vi "Add Annotation (by index).vi"(0 "FSM in":refnum<class "FSM.Graph.lvclass">, 5 "selectedEdge":i32, 7 "Name":string, 9 "Style":T1, 11 "error in (no error)":errorcluster) -> (4 "FSM out":refnum<class "FSM.Graph.lvclass">, 6 "Changed?":bool, 15 "error out":errorcluster)   [LabVIEW 2015, in "FSM.Graph.lvclass"]
uses:
  FSM.Graph.lvclass
  FSM.Annotation/Annotation Style.ctl
  FSM.Graph.lvclass/FSM.Graph.ctl
  FSM.Edge/FSM.Edge.lvclass
  FSM.Annotation/FSM.Annotation.lvclass
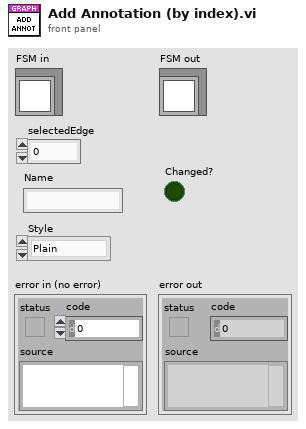
[diagram p1: front panel]
types:
  T1 = typedef "FSM.Annotation.lvclass/Annotation Style.ctl" = enum16{"Plain", "On", "Off", "On-Off"}
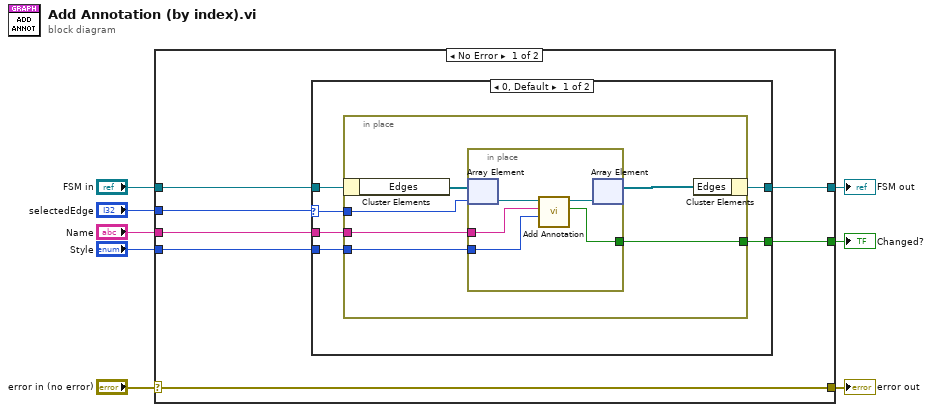
[diagram p0: block diagram]
diagram:
  n1 = case shown="No Error" "error in (no error)" {
    selector: "error in (no error)" -> [w15 w35]
    tunnel: [w15 w35] -> w7
    tunnel: [w13 w34] -> w5
    tunnel: "FSM in" -> [w14 w34]
    tunnel: "Name" -> [w12 _]
    tunnel: "Style" -> [w11 _]
    tunnel: [w10 _] -> w2
    tunnel: "selectedEdge" -> [w9 _]
    frame No Error {
      n2 = case shown="0, Default" w9 {
        selector: w9 -> [w20 _]
        tunnel: w14 -> [w21 w33]
        tunnel: [w17 w33] -> w13
        tunnel: w12 -> [w19 _]
        tunnel: w11 -> [w18 _]
        tunnel: [w16 _] -> w10
        frame 0, Default {
          n3 = in-place {
            in-place-border: w20 -> [w26]
            in-place-border: w19 -> [w25]
            in-place-border: w18 -> [w24]
            in-place-border: [w22] -> w16
            n4 = in-place-cluster #1(w21) -> ("Edges"=w27:refnum<class "FSM.Edge.lvclass">[])
            n5 = in-place {
              in-place-border: w25 -> [w30]
              in-place-border: w24 -> [w29]
              in-place-border: [w28] -> w22
              n6 = in-place-array #2(w27, w26) -> (w32:refnum<class "FSM.Edge.lvclass">)
              n7 = call "Add Annotation.vi"("Style"=w29, "Name"=w30, "FSM.Edge in"=w32) -> ("Changed?"=w28:bool, "FSM.Edge out"=w31:refnum<class "FSM.Edge.lvclass">)  [unwired: 6 in, 1 out]
              n8 = in-place-array #2(w31) -> (w23:refnum<class "FSM.Edge.lvclass">[])  [unwired: 1 out]
            }
            n9 = in-place-cluster #1("Edges"=w23) -> (w17:refnum<class "FSM.Graph.lvclass">)
          }
        }
        frame -1 {
        }
      }
    }
    frame Error {
    }
  }
  "error out" <- w7
  "FSM out" <- w5
  "Changed?" <- w2
